vi "Update Plots for Spectra Graph.vi"(0 "Spectral Data":T2={"PDT Amp [v]"=0.0, "RIS Amp [v]"=0.0, "B-Field"=[], "All In-Phase Scan Spectra"=[], "Model Select"=enum."OneCompRISTwoPDT", "Fit Each Scan"=FALSE, "PDT Center [g]"=0.0, "In-Phase Average Spectra"=[], "In-Phase Median Spectra"=[], "Out-Phase Median Spectra"=[], "Out-Phase Average Spectra"=[], "Fit Spectra"=[], "Fit No-Baseline Spectra"=[], "All Out-Phase Scan Spectra"=[], "Baseline Offset Correction"=FALSE, "In-Phase Offset [v]"=0.0, "Out-Phase Offset [v]"=0.0, "Ch2 Input\n(Balance)"=[], "Ch3 Input\n(Phase)"=[], "Ch4 Input\n(AFC)"=[], "Fit Pars"=[], "Fit Pars Errors"=[], "Fit Pars Labels"=[], "Raw Scan DAQ Data"=[], "Bad Scans Indicies"=[], "Good In-Phase Scan Spectra"=[], "Good Out-Phase Scan Spectra"=[], "Bad In-Phase Scan Spectra"=[], "Bad Out-Phase Scan Spectra"=[], "Number of bad scans"=0, "Fit History"=[], "PDT Amp. History/Set [v]"=[], "RIS Amp. History/Set [v]"=[], "RIS Amp. History/Scan [v]"=[], "All Shifted B-Fields"=[], "Good Shifted B-Fields"=[], "Ch5 Input\n(SpO2)"=[], "Ch6 Input\n(BPM)"=[], "Global SNR"=0.0, "Fit Error History"=[], "SNR History"=[]} {"Global SNR" min=0.0; "PDT Center [g]" min=0.0; "RIS Amp [v]" min=0.0}, 1 "Acquisition Parameters":T1={"Magnet Angle [deg]"=0.0, "Magnet Angles [deg]"=[], "DeltaVpp [v]"=0.0, "SEM [v]"=0.0, "DeltaVpp Thresh [v]"=0.0, "SEM Thresh [v]"=0.0, "Adaptive Processing"=FALSE, "Acquire Q"=FALSE, "Acquire Photos"=FALSE, "Adaptive Tuning"=FALSE, "Automated Matching"=FALSE, "X-Gradient [G/mm]"=0.0, "Y-Gradient [G/mm]"=0.0, "Z-Gradient [G/mm]"=0.0, "Central Field [G]"=0.0, "Scan Width [G]"=0.0, "Mod. Amp. [G]"=0.0, "Scan Time [s]"=0.0, "Pre-Scan Delay [ms]"=0, "Measurement Timeout [s]"=0.0, "Electromagnet Main Field [G]"=0.0, "Locked Central Field [G]"=0.0, "Scans Excluded"=0, "Scans Completed"=0, "No. Scans/Set"=0, "No. Scans for SNR"=0, "Field Locked Frequency [GHz]"=0.0, "Auto Set-based Field Center"=FALSE, "Prompt for oxy acquisition updates"=FALSE, "Oxy QA Scan?"=FALSE, "Exclude Bad Data"=FALSE, "Optimizing RF Power"=FALSE, "Gradients on/off"=TRUE, "Running Script"=FALSE, "Opto-Coupler Current [A]"=0.0, "Continuous Sweeping"=FALSE, "Sweep Rise Time [sec]"=0, "Reverse Sweep Central Field [G]"=0.0, "Forward Sweep Central Field [G]"=0.0, "Sweep Calibrated"=FALSE, "Modulation Calibrated"=FALSE, "First CheckCal Scan?"=FALSE, "AFC Field Correction"=FALSE, "OxyQAInit Scan Width [G]"=0.0, "OxyQAInit Mod. Amp. [G]"=0.0, "Scans Completed/Session"=0, "Acquire SpO2"=FALSE, "Acquire Temperature"=FALSE, "Over Mod"=FALSE} {"OxyQAInit Mod. Amp. [G]" min=0.0; "OxyQAInit Scan Width [G]" min=0.0; "Mod. Amp. [G]" min=0.0; "Scan Width [G]" min=0.0; "Measurement Timeout [s]" min=0.0; "Scan Time [s]" min=0.0; "Z-Gradient [G/mm]" min=0.0; "Y-Gradient [G/mm]" min=0.0; "X-Gradient [G/mm]" min=0.0; "SEM Thresh [v]" min=0.0; "DeltaVpp Thresh [v]" min=0.0; "SEM [v]" min=0.0}) -> ()   [LabVIEW 2016]
uses:
  Types/Spectral Data.ctl
  Types/Fitting Model Selection.ctl
  Types/Acquisition Parameters.ctl
  Types/Global Variables.vi
panel:
  # "Gradients"
  # "Field"
  # "Scans and Sets"
  # "Timing"
  # "Adaptive Dosimetric \nData Processing"
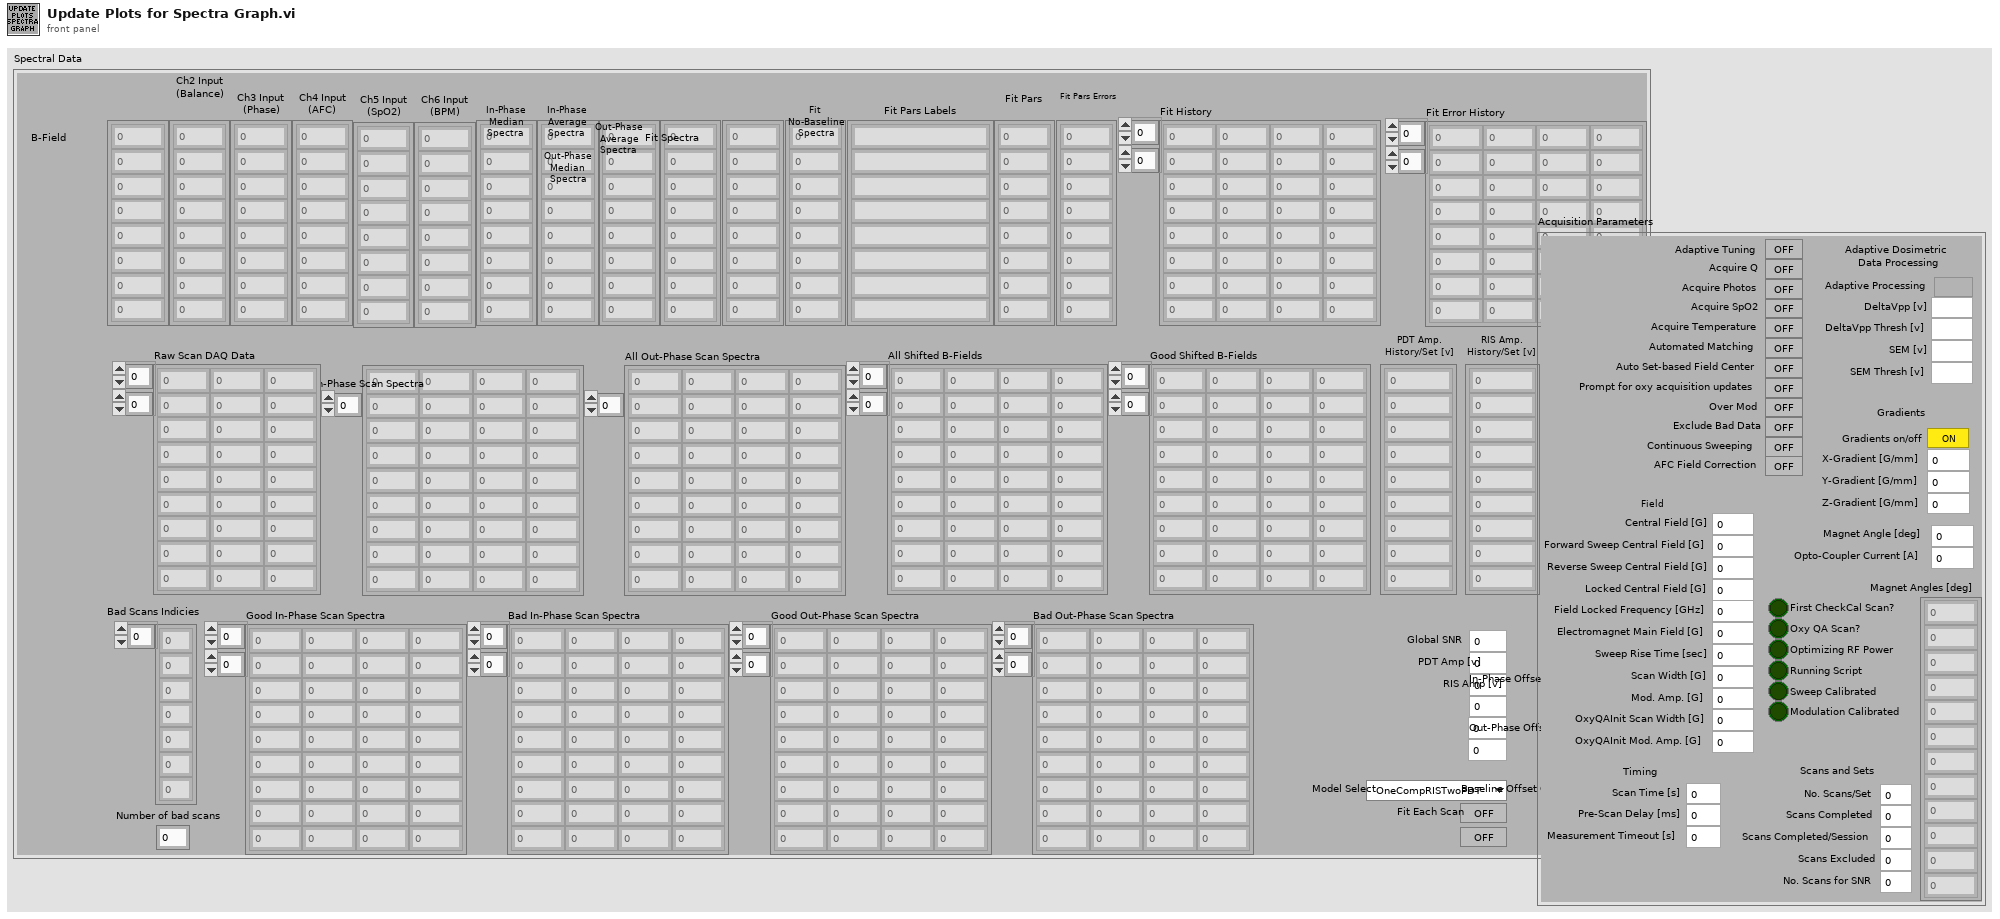
[diagram p1: front panel]
types:
  T1 = typedef "Acquisition Parameters.ctl" = cluster{"Magnet Angle [deg]":dbl, "Magnet Angles [deg]":dbl[], "DeltaVpp [v]":dbl, "SEM [v]":dbl, "DeltaVpp Thresh [v]":dbl, "SEM Thresh [v]":dbl, "Adaptive Processing":bool, "Acquire Q":bool, "Acquire Photos":bool, "Adaptive Tuning":bool, "Automated Matching":bool, "X-Gradient [G/mm]":dbl, "Y-Gradient [G/mm]":dbl, "Z-Gradient [G/mm]":dbl, "Central Field [G]":dbl, "Scan Width [G]":dbl, "Mod. Amp. [G]":dbl, "Scan Time [s]":dbl, "Pre-Scan Delay [ms]":u32, "Measurement Timeout [s]":dbl, "Electromagnet Main Field [G]":dbl, "Locked Central Field [G]":dbl, "Scans Excluded":u32, "Scans Completed":u32, "No. Scans/Set":u32, "No. Scans for SNR":u32, "Field Locked Frequency [GHz]":dbl, "Auto Set-based Field Center":bool, "Prompt for oxy acquisition updates":bool, "Oxy QA Scan?":bool, "Exclude Bad Data":bool, "Optimizing RF Power":bool, "Gradients on/off":bool, "Running Script":bool, "Opto-Coupler Current [A]":dbl, "Continuous Sweeping":bool, "Sweep Rise Time [sec]":u32, "Reverse Sweep Central Field [G]":dbl, "Forward Sweep Central Field [G]":dbl, "Sweep Calibrated":bool, "Modulation Calibrated":bool, "First CheckCal Scan?":bool, "AFC Field Correction":bool, "OxyQAInit Scan Width [G]":dbl, "OxyQAInit Mod. Amp. [G]":dbl, "Scans Completed/Session":u32, "Acquire SpO2":bool, "Acquire Temperature":bool, "Over Mod":bool}
  T2 = typedef "Spectral Data.ctl" = cluster{"PDT Amp [v]":dbl, "RIS Amp [v]":dbl, "B-Field":dbl[], "All In-Phase Scan Spectra":dbl[][], "Model Select":T3, "Fit Each Scan":bool, "PDT Center [g]":dbl, "In-Phase Average Spectra":dbl[], "In-Phase Median Spectra":dbl[], "Out-Phase Median Spectra":dbl[], "Out-Phase Average Spectra":dbl[], "Fit Spectra":dbl[], "Fit No-Baseline Spectra":dbl[], "All Out-Phase Scan Spectra":dbl[][], "Baseline Offset Correction":bool, "In-Phase Offset [v]":dbl, "Out-Phase Offset [v]":dbl, "Ch2 Input\n(Balance)":dbl[], "Ch3 Input\n(Phase)":dbl[], "Ch4 Input\n(AFC)":dbl[], "Fit Pars":dbl[], "Fit Pars Errors":dbl[], "Fit Pars Labels":string[], "Raw Scan DAQ Data":dbl[][], "Bad Scans Indicies":i32[], "Good In-Phase Scan Spectra":dbl[][], "Good Out-Phase Scan Spectra":dbl[][], "Bad In-Phase Scan Spectra":dbl[][], "Bad Out-Phase Scan Spectra":dbl[][], "Number of bad scans":i32, "Fit History":dbl[][], "PDT Amp. History/Set [v]":dbl[], "RIS Amp. History/Set [v]":dbl[], "RIS Amp. History/Scan [v]":dbl[], "All Shifted B-Fields":dbl[][], "Good Shifted B-Fields":dbl[][], "Ch5 Input\n(SpO2)":dbl[], "Ch6 Input\n(BPM)":dbl[], "Global SNR":dbl, "Fit Error History":dbl[][], "SNR History":dbl[]}
  T3 = typedef "Fitting Model Selection.ctl" = enum16{"OneCompRIS", "OneCompRISTwoPDT", "OneCompRISRev", "OneCompRISTwoPDTRev", "LiPc", "TwoLiPc", "ThreeLiPc", "FourLiPc", "PDTCalibration", "CE_Ink", "Printex", "MelaninTwoPDT"}
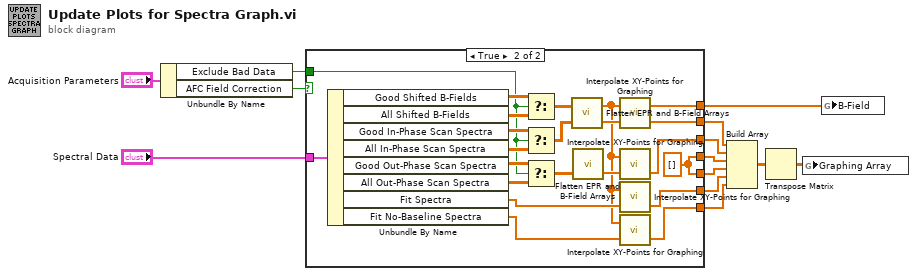
[diagram p0: block diagram]
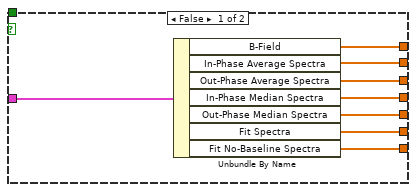
[diagram p2: hidden frame]
diagram:
  n1 = Unbundle By Name("Acquisition Parameters") -> ("Exclude Bad Data"=w1:bool, "AFC Field Correction"=w2:bool)
  n2 = case shown="True" w2 {
    tunnel: [w21 w28] -> w13
    tunnel: [w20 w32] -> w12
    tunnel: [w19 w32] -> w11
    tunnel: [w18 w29] -> w8
    tunnel: "Spectral Data" -> [w17 w34]
    tunnel: [w16 w25] -> w6
    tunnel: [w15 w22] -> w5
    tunnel: [w14 w30] -> w4
    tunnel: w1 -> [_ w33]
    frame False {
      n3 = Unbundle By Name(w17) -> ("B-Field"=w14:dbl[], "In-Phase Average Spectra"=w18:dbl[], "Out-Phase Average Spectra"=w21:dbl[], "In-Phase Median Spectra"=w20:dbl[], "Out-Phase Median Spectra"=w19:dbl[], "Fit Spectra"=w16:dbl[], "Fit No-Baseline Spectra"=w15:dbl[])
    }
    frame True {
      w32 = dbl[] [] ("In-Phase Median Spectra")
      n4 = Unbundle By Name(w34) -> ("Good Shifted B-Fields"=w35:dbl[][], "All Shifted B-Fields"=w36:dbl[][], "Good In-Phase Scan Spectra"=w37:dbl[][], "All In-Phase Scan Spectra"=w38:dbl[][], "Good Out-Phase Scan Spectra"=w39:dbl[][], "All Out-Phase Scan Spectra"=w40:dbl[][], "Fit Spectra"=w26:dbl[], "Fit No-Baseline Spectra"=w24:dbl[])
      n5 = Select(t=w35, s=w33, f=w36) -> (s? t:f=w42:dbl[][])
      n6 = Select(t=w37, s=w33, f=w38) -> (s? t:f=w41:dbl[][])
      n7 = Select(t=w39, s=w33, f=w40) -> (s? t:f=w43:dbl[][])
      n8 = call "Flatten EPR and B-Field Arrays.vi"("2D EPR Data"=w41, "2D B-Fields"=w42) -> ("1D Flattened EPR Data"=w31:dbl[], "1D Flattened B-Fields"=w23:dbl[])
      n9 = call "Flatten EPR and B-Field Arrays.vi"("2D EPR Data"=w43) -> ("1D Flattened EPR Data"=w27:dbl[])  [unwired: 1 in, 1 out]
      n10 = call "Interpolate XY-Points for Graphing.vi"("Y"=w31, "X"=w23) -> ("Y-Interpolated"=w29:dbl[], "X-Interpolated"=w30:dbl[])
      n11 = call "Interpolate XY-Points for Graphing.vi"("Y"=w27, "X"=w23) -> ("Y-Interpolated"=w28:dbl[])  [unwired: 1 out]
      n12 = call "Interpolate XY-Points for Graphing.vi"("Y"=w26, "X"=w23) -> ("Y-Interpolated"=w25:dbl[])  [unwired: 1 out]
      n13 = call "Interpolate XY-Points for Graphing.vi"("Y"=w24, "X"=w23) -> ("Y-Interpolated"=w22:dbl[])  [unwired: 1 out]
    }
  }
  n14 = Build Array(w8, w13, w12, w11, w6, w5) -> (w10:dbl[][])
  n15 = Transpose Matrix(1:w10) -> (0:w9:dbl[][])
  n16 = global write "Global Variables.vi" "Graphing Array"(w9) -> ()
  n17 = global write "Global Variables.vi" "B-Field"(w4) -> ()
